vi "CheckDwellTime.vi"(10 "trigger in":bool, 11 "condition in":T1) -> (1 "updated":bool, 2 "trigger out":bool, 3 "condition out":T1)   [LabVIEW 2017, in "Trigger.lvlib"]
uses:
  <vilib>/addons/InsightCM/Devices/Shared/Common/Trigger/Trigger.lvlib
  <vilib>/addons/InsightCM/Devices/Shared/Common/Trigger/controls/TriggerCondition.ctl
  <vilib>/addons/InsightCM/MessageBus/Base/controls/Condition.ctl
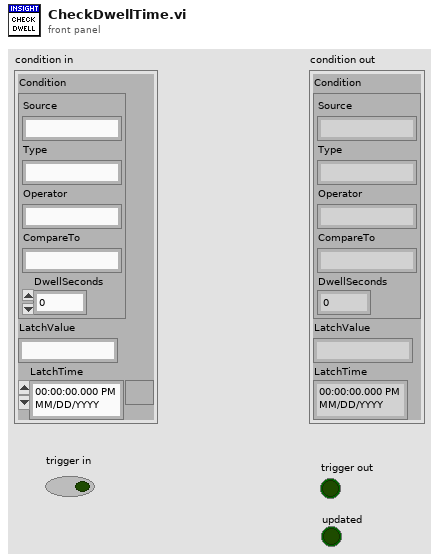
[diagram p1: front panel]
types:
  T1 = typedef "Trigger.lvlib/TriggerCondition.ctl" = cluster{"Condition":T2, "LatchValue":string, "LatchTime":timestamp}
  T2 = typedef "Condition.ctl" = cluster{"Source":string, "Type":string, "Operator":string, "CompareTo":string, "DwellSeconds":dbl}
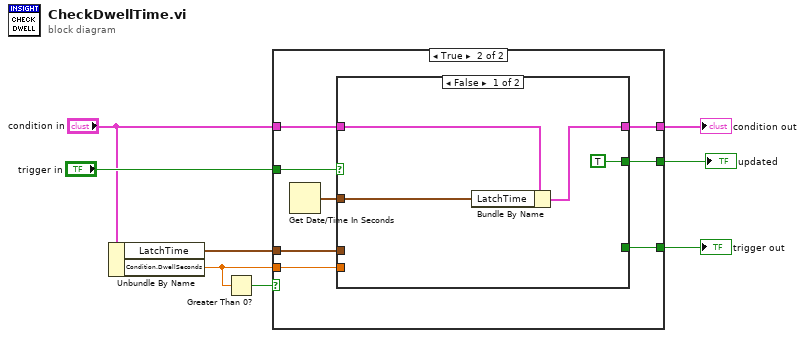
[diagram p0: block diagram]
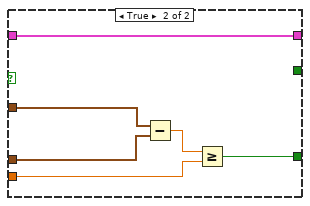
[diagram p3: hidden frame]
diagram:
  n1 = Unbundle By Name("condition in") -> ("LatchTime"=w4:timestamp, "Condition.DwellSeconds"=w3:dbl)
  n2 = Greater Than 0?(x=w3) -> (x > 0?=w2:bool)
  n3 = case shown="True" w2 {
    tunnel: [w10 w18] -> w8
    tunnel: [w9 w17] -> w7
    tunnel: "trigger in" -> [w10 w16]
    tunnel: "condition in" -> [w9 w14]
    tunnel: w4 -> [_ w13]
    tunnel: w3 -> [_ w12]
    tunnel: [_ w11] -> w1
    frame False {
    }
    frame True {
      n4 = Get Date/Time In Seconds() -> (seconds since 1Jan1904=w15:timestamp)
      n5 = case shown="False" w16 {
        tunnel: [_ w25] -> w18
        tunnel: w14 -> [w22 w26]
        tunnel: [w21 w26] -> w17
        tunnel: w15 -> [w20 w27]
        tunnel: w13 -> [_ w24]
        tunnel: w12 -> [_ w23]
        tunnel: [TRUE _] -> w11
        frame False {
          n6 = Bundle By Name(cluster=w22, "LatchTime"=w20) -> (w21:T1)
        }
        frame True {
          n7 = Subtract(x=w27, y=w24) -> (x-y=w28:dbl)
          n8 = Greater Or Equal?(x=w28, y=w23) -> (x >= y?=w25:bool)
        }
      }
    }
  }
  "condition out" <- w7
  "trigger out" <- w8
  "updated" <- w1
